vi "Chi2 MLE.vi"(9 "f(X)":dbl[](array[numeric]), 11 "Y":dbl[](array[numeric])) -> (3 "chi2_mle":dbl)   [LabVIEW 2021, in "Fits.lvlib"]
uses:
  Fits.lvlib
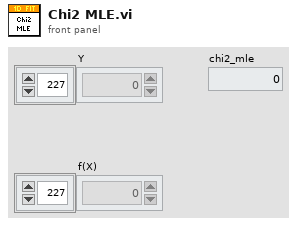
[diagram p1: front panel]
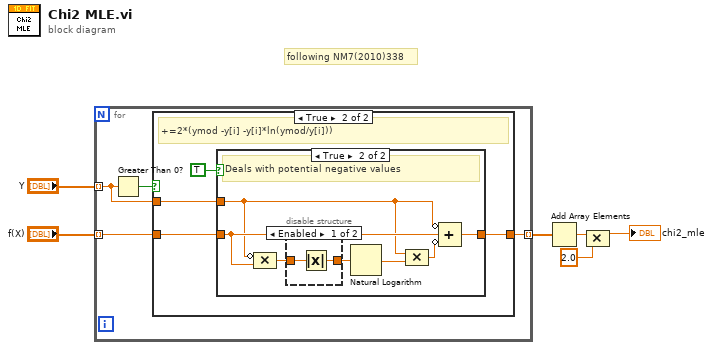
[diagram p0: block diagram]
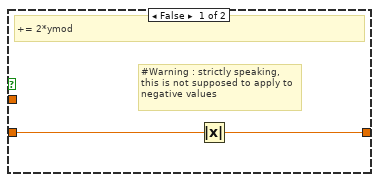
[diagram p2: hidden frame]
diagram:
  # "following NM7(2010)338"
  n1 = for {
    tunnel: "f(X)" -> [w9] mode=indexing
    tunnel: "Y" -> [w7] mode=indexing
    tunnel: [w8] -> w4 mode=indexing
    n2 = Greater Than 0?(x=w7) -> (x > 0?=w10:bool)
    n3 = case shown="True" w10 {
      tunnel: w9 -> [w12 w14]
      tunnel: [w11 w16] -> w8
      tunnel: w7 -> [_ w15]
      frame False {
        # "#Warning : strictly speaking, this is not supposed to apply to negative values"
        # "+= 2*ymod"
        n4 = Absolute Value(x=w12) -> (abs(x)=w11:dbl)
      }
      frame True {
        # "+=2*(ymod -y[i] -y[i]*ln(ymod/y[i]))"
        n5 = case shown="True" TRUE {
          tunnel: [_ w23] -> w16
          tunnel: w14 -> [_ w22]
          tunnel: w15 -> [_ w20]
          frame False {
          }
          frame True {
            # "Deals with potential negative values"
            n6 = Compound Arithmetic op=MULTIPLY(invert w20, w22) -> (w21:dbl)
            n7 = disable-structure shown="Enabled" {
              disable-tunnel: w21 -> [w25 w26]
              disable-tunnel: [w24 w26] -> w17
              frame Enabled {
                n8 = Absolute Value(x=w25) -> (abs(x)=w24:dbl)
              }
              frame Disabled {
              }
            }
            n9 = Natural Logarithm(1:w17) -> (0:w19:dbl)
            n10 = Compound Arithmetic op=MULTIPLY(w20, w19) -> (w18:dbl)
            n11 = Compound Arithmetic op=ADD(invert w20, w22, invert w18) -> (w23:dbl)
          }
        }
      }
    }
  }
  n12 = Add Array Elements(numeric array=w4) -> (sum=w3:dbl)
  n13 = Compound Arithmetic op=MULTIPLY(w3, 2.0 ("value")) -> (→"chi2_mle":dbl)
